vi "Copy Keys (recursive).vi"(7 "Root Node in":variant, 8 "error in":errorcluster, 10 "Section":string, 11 "Additional Config":refnum<class "config-base.lvclass">) -> (0 "error out":errorcluster, 5 "Root Node out":variant)   [LabVIEW 2020, in "hse-config.lvlib" / "config-base.lvclass"]
doc: "Copies all keys from the given Additional Config recursively into the Root Node.\n\n____\nHAMPEL SOFTWARE ENGINEERING v3.8.0 (2023-12-18 14:41)"
uses:
  config-base.lvclass
  config-base.lvclass/config-base.ctl
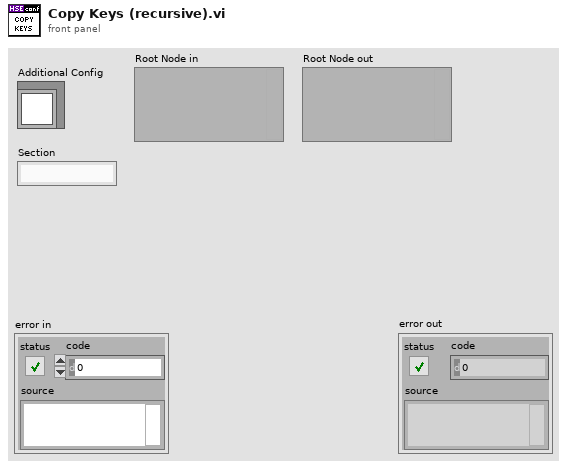
[diagram p1: front panel]
types:
  T1 = typedef "NI_Data Type.lvlib/Data Type.ctl" = enum8{"Invalid Type", "Void", "I8", "I16", "I32", "I64", "U8", "U16", "U32", "U64", "Single Float", "Double Float", "Extended Float", "Single Complex", "Double Complex", "Extended Complex", "Enum U8", "Enum U16", "Enum U32", "Enum U64", "Single Float With Unit", "Double Float With Unit", "Extended Float With Unit", "Single Complex with Unit", "Double Complex with Unit", "Extended Complex with Unit", "Boolean", "String", "Path", "Picture", "Tag", "Array", "Cluster", "Variant", "LV Variant", "Waveform", "Timestamp", "Digital Waveform", "Digital Data", "ExpressData", "Refnum", "External Data", "VI", "Poly VI", "LabVIEW Class Instance", "Fixed Point", "Set Collection", "Map Collection"}
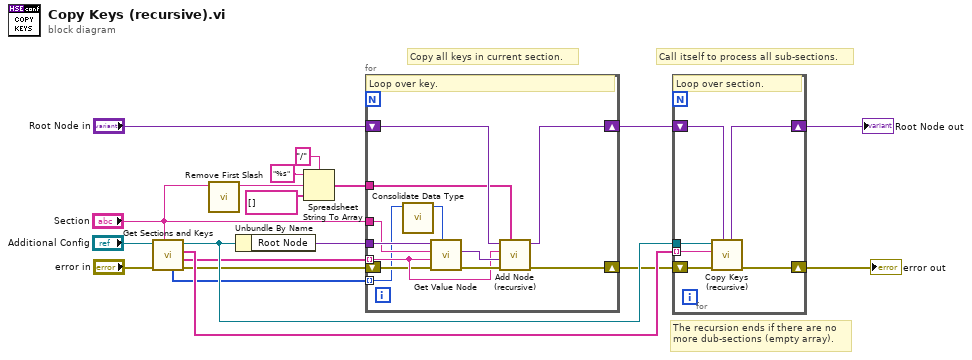
[diagram p0: block diagram]
diagram:
  # "The recursion ends if there are no\nmore dub-sections (empty array)."
  # "Call itself to process all sub-sections."
  # "Copy all keys in current section."
  n1 = call-dynamic "Get Sections and Keys.vi"("Section"="Section", "error in"="error in", "config-base in"="Additional Config") -> ("error out"=w8:errorcluster, "Keys"=w7:string[], "Sections"=w17:string[], "config-base out"=w19:refnum<class "config-base.lvclass">, "Key Data Types"=w10:T1[])  [unwired: 4 in]
  n2 = call "Remove First Slash.vi"("Section"="Section") -> ("result string"=w14:string)  [unwired: 10 in]
  n3 = Unbundle By Name(w19) -> ("Root Node"=w18:variant)
  n4 = Spreadsheet String To Array(delimiter (Tab)="/" ("Split Pattern"), format string="%s", spreadsheet string=w14, array type (2D Dbl)=string[] []) -> (array=w16:string[])
  n5 = for {
    tunnel: w7 -> [w29] mode=indexing
    shift-right: [w22] -> w4
    shift-left: w8 -> [w26]
    tunnel: "Section" -> [w25]
    shift-right: [w23] -> w2
    shift-left: "Root Node in" -> [w28]
    tunnel: w18 -> [w27]
    tunnel: w10 -> [w21] mode=indexing
    tunnel: w16 -> [w24]
    # "Loop over key."
    n6 = call "Consolidate Data Type.vi"("Type in"=w21) -> ("Type out"=w20:T1)  [unwired: 10 in]
    n7 = call "Get Value Node.vi"("Data Type"=w20, "error in"=w26, "Key"=w29, "Section"=w25, "Root Node"=w27) -> ("error out"=w31:errorcluster, "Value Node out"=w30:variant)  [unwired: 5 in]
    n8 = call "Add Node (recursive).vi"("Section"=w24, "error in"=w31, "Value"=w30, "Key"=w29, "Node in"=w28) -> ("error out"=w22:errorcluster, "Node out"=w23:variant)  [unwired: 5 in]
  }
  n9 = for {
    tunnel: w17 -> [w36] mode=indexing
    shift-right: [w32] -> w3
    shift-left: w4 -> [w37]
    tunnel: w19 -> [w35]
    shift-right: [w33] -> w1
    shift-left: w2 -> [w34]
    # "Loop over section."
    n10 = call "Copy Keys (recursive).vi"("Root Node in"=w34, "error in"=w37, "Section"=w36, "Additional Config"=w35) -> ("error out"=w32:errorcluster, "Root Node out"=w33:variant)  [unwired: 6 in]
  }
  "error out" <- w3
  "Root Node out" <- w1
